vi "test - Convert config array - Boolean - 1.vi"(8 "error in (no error)":errorcluster, 11 "TestCase in":refnum<class "Create New Assert Tester.lvclass">) -> (0 "error out":errorcluster, 3 "TestCase out":refnum<class "Create New Assert Tester.lvclass">)   [LabVIEW 2017, in "Create New Assert Tester.lvclass"]
uses:
  Create New Assert Tester.lvclass
  Plugins/Utility/Assert Build Configuration.ctl
  Core/Assert API Components/Failure Actions.ctl
  <vilib>/Utility/Data Type/Type Definitions/Data Type.ctl
  Plugins/Utility/Assert Scripting Configuration.ctl
  <vilib>/addons/_JKI Toolkits/VI Tester/TestCase.llb/TestCase.lvclass
  <vilib>/Utility/Data Type/NI_Data Type.lvlib
  Core/Assert API Components/Assert API Components.lvlib
  C:/Program Files (x86)/National Instruments/LabVIEW 2017/vi.lib/addons/_JKI Toolkits/VI Tester/TestCase.llb/TestCase.lvclass
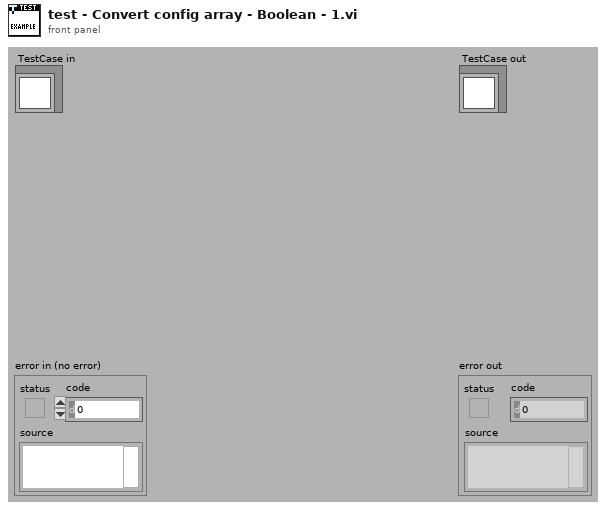
[diagram p1: front panel]
types:
  T1 = typedef "Assert Build Configuration.ctl" = cluster{"Assert Name":string, "Operation":string, "Comparison Value 1":string, "Comparison Value 2":string, "Comment":string, "Default Failure Action":T2, "Description":string, "Operation Display":string, "Active":bool, "Data Type":T3}
  T2 = typedef "Assert API Components.lvlib/Failure Actions.ctl" = enum16{"None", "Log To File", "Pause Execution", "Abort Execution"}
  T3 = typedef "NI_Data Type.lvlib/Data Type.ctl" = enum8{"Invalid Type", "Void", "I8", "I16", "I32", "I64", "U8", "U16", "U32", "U64", "Single Float", "Double Float", "Extended Float", "Single Complex", "Double Complex", "Extended Complex", "Enum U8", "Enum U16", "Enum U32", "Enum U64", "Single Float With Unit", "Double Float With Unit", "Extended Float With Unit", "Single Complex with Unit", "Double Complex with Unit", "Extended Complex with Unit", "Boolean", "String", "Path", "Picture", "Tag", "Array", "Cluster", "Variant", "LV Variant", "Waveform", "Timestamp", "Digital Waveform", "Digital Data", "ExpressData", "Refnum", "External Data", "VI", "Poly VI", "LabVIEW Class Instance", "Fixed Point"}
  T4 = enum16{"None", "Log To File", "Pause Execution", "Abort Execution"}
  T5 = typedef "Assert Scripting Configuration.ctl" = cluster{"Assert Name":string, "Comment":string, "Numeric Operation":string, "Type":T3, "String Operation":string, "DBL Comparison Value 1":dbl, "DBL Comparison Value 2":dbl, "I32 Comparison Value 1":i32, "I32 Comparison Value 2":i32, "Creator":string, "Creation Timestamp":timestamp, "String Comparison Value":string, "Description":string, "Default Failure Action":enum16{"None", "Log To File", "Pause Execution", "Abort Execution"}, "Boolean Comparison Value":bool, "I8 Comparison Value 1":i8, "I8 Comparison Value 2":i8, "I16 Comparison Value 1":i16, "I16 Comparison Value 2":i16, "I64 Comparison Value 1":i64, "I64 Comparison Value 2":i64, "U8 Comparison Value 1":u8, "U8 Comparison Value 2":u8, "U16 Comparison Value 1":u16, "U16 Comparison Value 2":u16, "U32 Comparison Value 1":u32, "U32 Comparison Value 2":u32, "U64 Comparison Value 1":u64, "U64 Comparison Value 2":u64, "EXT Comparison Value 1":ext, "EXT Comparison Value 2":ext, "SGL Comparison Value 1":sgl, "SGL Comparison Value 2":sgl, "Float Digits of Precision":u8}
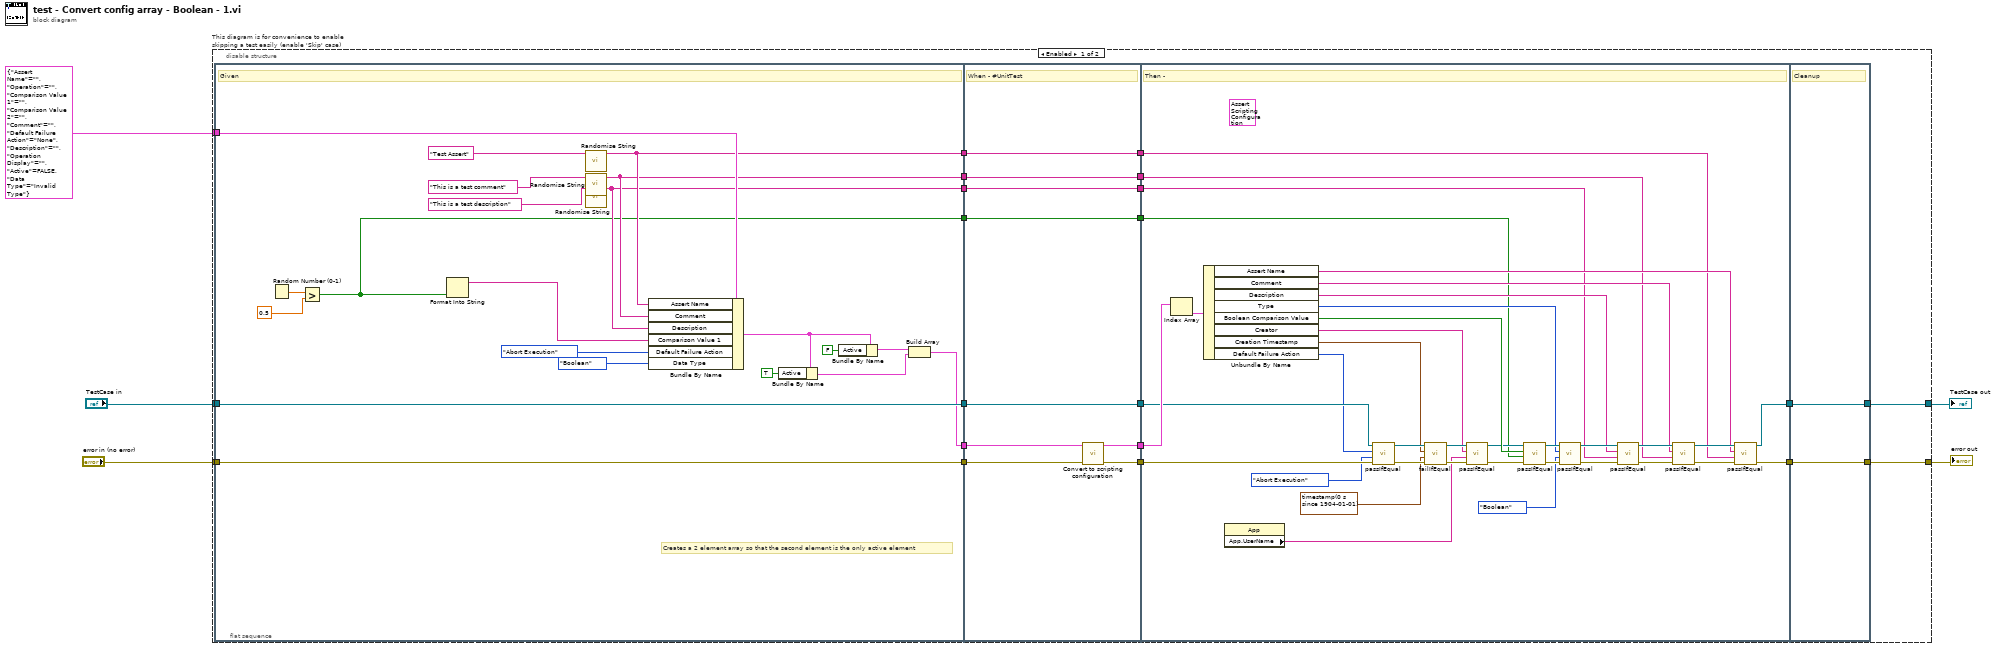
[diagram p0: block diagram]
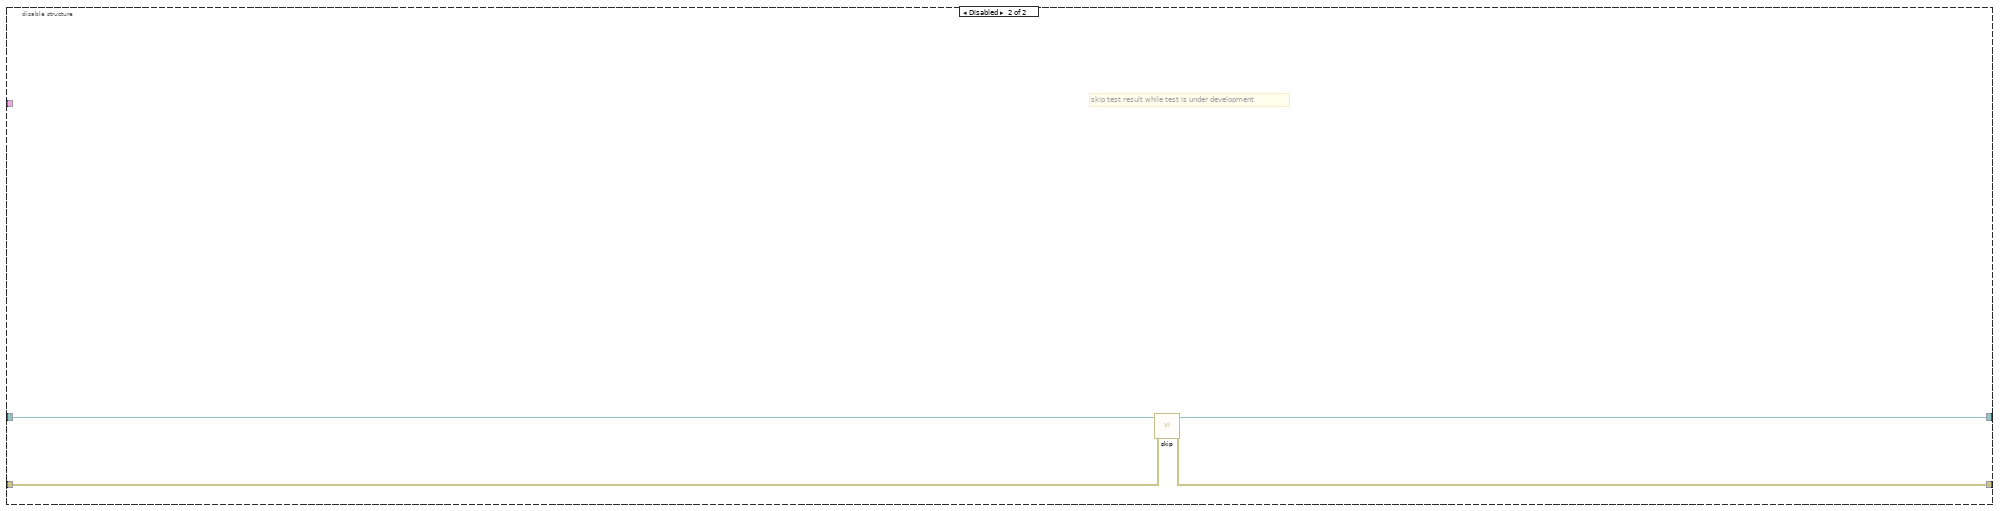
[diagram p2: hidden frame]
diagram:
  n1 = disable-structure "This diagram is for convenience to enable skipping a test easily (enable 'Skip' case)" shown="Enabled" {
    disable-tunnel: "TestCase in" -> [w20 w98]
    disable-tunnel: [w17 w96] -> w2
    disable-tunnel: [w18 w97] -> w4
    disable-tunnel: "error in (no error)" -> [w19 w95]
    disable-tunnel: T1 {"Assert Name"="", "Operation"="", "Comparison Value 1"="", "Comparison Value 2"="", "Comment"="", "Default Failure Action"=enum."None", "Description"="", "Operation Display"="", "Active"=FALSE, "Data Type"=enum."Invalid Type"} ("Assert Build Configuration") -> [w15 _]
    frame Enabled {
      n2 = flat-sequence {
        tunnel: w19 -> [w46]
        tunnel: w20 -> [w47]
        tunnel: [w47] -> w26
        tunnel: [w46] -> w25
        tunnel: w15 -> [w45]
        tunnel: [w41] -> w14
        tunnel: [w33] -> w12
        tunnel: [w32] -> w10
        tunnel: [w31] -> w8
        tunnel: [w27] -> w6
        tunnel: [w56] -> w24
        tunnel: [w54] -> w23
        tunnel: w26 -> [w56]
        tunnel: w25 -> [w55]
        tunnel: [w53] -> w16
        tunnel: w14 -> [w52]
        tunnel: [w51] -> w13
        tunnel: w12 -> [w51]
        tunnel: [w50] -> w11
        tunnel: w10 -> [w50]
        tunnel: [w49] -> w9
        tunnel: w8 -> [w49]
        tunnel: [w48] -> w7
        tunnel: w6 -> [w48]
        tunnel: [w63] -> w22
        tunnel: [w64] -> w21
        tunnel: w24 -> [w87]
        tunnel: w23 -> [w92]
        tunnel: w16 -> [w90]
        tunnel: w13 -> [w59]
        tunnel: w11 -> [w60]
        tunnel: w9 -> [w61]
        tunnel: w7 -> [w57]
        tunnel: [w93] -> w18
        tunnel: [w94] -> w17
        tunnel: w22 -> [w94]
        tunnel: w21 -> [w93]
        frame #0 {
          # "Creates a 2 element array so that the second element is the only active element"
          # "Given"
          n3 = Random Number (0-1)() -> (number: 0 to 1=w30:dbl)
          n4 = Greater?(x=w30, y=0.5 ("x")) -> (0:w27:bool)
          n5 = Format Into String(w27) -> (resulting string=w28:string)  [unwired: 3 in, 1 out]
          n6 = call "Randomise String.vi"("String in"="Test Assert" ("Assert Name")) -> ("String out"=w33:string)  [unwired: 10 in]
          n7 = call "Randomise String.vi"("String in"="This is a test comment" ("Comment")) -> ("String out"=w32:string)  [unwired: 10 in]
          n8 = call "Randomise String.vi"("String in"="This is a test description" ("Comment")) -> ("String out"=w31:string)  [unwired: 10 in]
          n9 = Bundle By Name(cluster=w45, "Assert Name"=w33, "Comment"=w32, "Description"=w31, "Comparison Value 1"=w28, "Default Failure Action"=Failure_Actions."Abort Execution", "Data Type"=Data_Type."Boolean") -> (w38:T1)
          n10 = Bundle By Name(cluster=w38, "Active"=TRUE) -> (w36:T1)
          n11 = Bundle By Name(cluster=w38, "Active"=FALSE) -> (w40:T1)
          n12 = Build Array(w40, w36) -> (w41:T1[])
        }
        frame #1 {
          # "When - #UnitTest"
          n13 = call "Convert to scripting configuration.vi"("error in (no error)"=w55, "Multiple Assert Configuration"=w52) -> ("error out"=w54:errorcluster, "Array"=w53:T5[])  [unwired: 7 in, 1 out]
        }
        frame #2 {
          (unwired) T5 {"Assert Name"="", "Comment"="", "Numeric Operation"="", "Type"=enum."Invalid Type", "String Operation"="", "DBL Comparison Value 1"=0.0, "DBL Comparison Value 2"=0.0, "I32 Comparison Value 1"=0, "I32 Comparison Value 2"=0, "Creator"="", "Creation Timestamp"=timestamp(0 s since 1904-01-01), "String Comparison Value"="", "Description"="", "Default Failure Action"=enum."None", "Boolean Comparison Value"=FALSE, "I8 Comparison Value 1"=0, "I8 Comparison Value 2"=0, "I16 Comparison Value 1"=0, "I16 Comparison Value 2"=0, "I64 Comparison Value 1"=0, "I64 Comparison Value 2"=0, "U8 Comparison Value 1"=0, "U8 Comparison Value 2"=0, "U16 Comparison Value 1"=0, "U16 Comparison Value 2"=0, "U32 Comparison Value 1"=0, "U32 Comparison Value 2"=0, "U64 Comparison Value 1"=0, "U64 Comparison Value 2"=0, "EXT Comparison Value 1"=0.0, "EXT Comparison Value 2"=0.0, "SGL Comparison Value 1"=0.0, "SGL Comparison Value 2"=0.0, "Float Digits of Precision"=0} ("Assert Scripting Configuration")
          # "Then -"
          n14 = Index Array(array=w90) -> (element=w89:T5)  [unwired: 1 in]
          n15 = Unbundle By Name(w89) -> ("Assert Name"=w62:string, "Comment"=w70:string, "Description"=w71:string, "Type"=w72:T3, "Boolean Comparison Value"=w79:bool, "Creator"=w80:string, "Creation Timestamp"=w68:timestamp, "Default Failure Action"=w85:T4)
          n16 = property class="App"() -> ("App.UserName"=w66:string)  [unwired: 2 in, 2 out]
          n17 = call-dynamic "passIfEqual.vi"("error in (no error)"=w92, "y"=T4."Abort Execution" ("Default Failure Action"), "x"=w85, "TestCase in"=w87) -> ("error out"=w88:errorcluster, "TestCase out"=w86:refnum<class "Create New Assert Tester.lvclass">)  [unwired: 6 in]
          n18 = call-dynamic "failIfEqual.vi"("error in (no error)"=w88, "y"=timestamp(0 s since 1904-01-01) ("Creation Timestamp"), "x"=w68, "TestCase in"=w86) -> ("error out"=w91:errorcluster, "TestCase out"=w83:refnum<class "Create New Assert Tester.lvclass">)  [unwired: 6 in]
          n19 = call-dynamic "passIfEqual.vi"("error in (no error)"=w91, "y"=w66, "x"=w80, "TestCase in"=w83) -> ("error out"=w84:errorcluster, "TestCase out"=w58:refnum<class "Create New Assert Tester.lvclass">)  [unwired: 6 in]
          n20 = call-dynamic "passIfEqual.vi"("error in (no error)"=w84, "y"=w57, "x"=w79, "TestCase in"=w58) -> ("error out"=w82:errorcluster, "TestCase out"=w77:refnum<class "Create New Assert Tester.lvclass">)  [unwired: 6 in]
          n21 = call-dynamic "passIfEqual.vi"("error in (no error)"=w82, "y"=Data_Type."Boolean" ("Data Type"), "x"=w72, "TestCase in"=w77) -> ("error out"=w78:errorcluster, "TestCase out"=w76:refnum<class "Create New Assert Tester.lvclass">)  [unwired: 6 in]
          n22 = call-dynamic "passIfEqual.vi"("error in (no error)"=w78, "y"=w61, "x"=w71, "TestCase in"=w76) -> ("error out"=w81:errorcluster, "TestCase out"=w74:refnum<class "Create New Assert Tester.lvclass">)  [unwired: 6 in]
          n23 = call-dynamic "passIfEqual.vi"("error in (no error)"=w81, "y"=w60, "x"=w70, "TestCase in"=w74) -> ("error out"=w75:errorcluster, "TestCase out"=w73:refnum<class "Create New Assert Tester.lvclass">)  [unwired: 6 in]
          n24 = call-dynamic "passIfEqual.vi"("error in (no error)"=w75, "y"=w59, "x"=w62, "TestCase in"=w73) -> ("error out"=w64:errorcluster, "TestCase out"=w63:refnum<class "Create New Assert Tester.lvclass">)  [unwired: 6 in]
        }
        frame #3 {
          # "Cleanup"
        }
      }
    }
    frame Disabled {
      # "skip test result while test is under development"
      n25 = call <vilib>:"skip.vi"("error in (no error)"=w95, "TestCase in"=w98) -> ("error out"=w97:errorcluster, "TestCase out"=w96:refnum<class "Create New Assert Tester.lvclass">)  [unwired: 8 in]
    }
  }
  "error out" <- w4
  "TestCase out" <- w2
